vi "AutoBall.vi"(7 "Drive Params":T1, 8 "PID Params":T2, 10 "Command Array":dbl[](array[numeric])) -> (2 "isFinished":bool)   [LabVIEW 2013]
uses:
  AutoDriveParams.ctl
  Drivetrain/Drivetrain Control.ctl
  Drivetrain/DT Mode.ctl
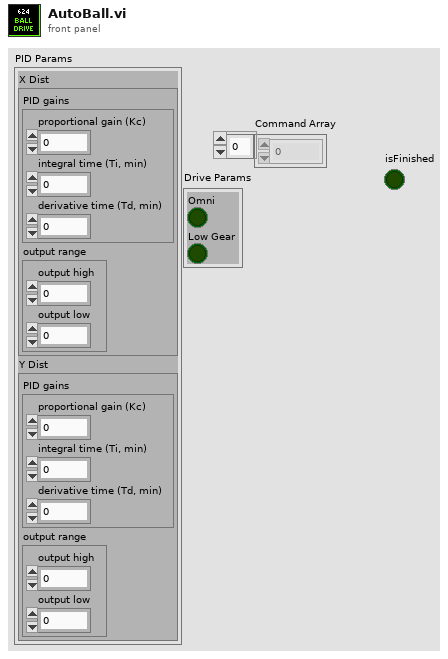
[diagram p1: front panel]
types:
  T1 = typedef "AutoDriveParams.ctl" = cluster{"Omni":bool, "Low Gear":bool}
  T2 = cluster{"X Dist":cluster{"PID gains":cluster{"proportional gain (Kc)":dbl, "integral time (Ti, min)":dbl, "derivative time (Td, min)":dbl}, "output range":cluster{"output high":dbl, "output low":dbl}}, "Y Dist":cluster{"PID gains":cluster{"proportional gain (Kc)":dbl, "integral time (Ti, min)":dbl, "derivative time (Td, min)":dbl}, "output range":cluster{"output high":dbl, "output low":dbl}}}
  T3 = typedef "DT Mode.ctl" = enum16{"Manual", "Gyro Steer", "Distance Drive", "Fieldcentric", "Roll Maneuver", "Alt Roll Maneuver"}
  T4 = typedef "Drivetrain Control.ctl" = cluster{"axis 1 (x)":dbl, "axis 2 (y)":dbl, "Mode":T3, "heading target":dbl, "steer axis":dbl, "omni?":bool, "Low Gear?":bool, "distance target":cluster{"x":dbl, "y":dbl}, "PID Params":cluster{"X Dist":cluster{"PID gains":cluster{"proportional gain (Kc)":dbl, "integral time (Ti, min)":dbl, "derivative time (Td, min)":dbl}, "output range":cluster{"output high":dbl, "output low":dbl}}, "Y Dist":cluster{"PID gains":cluster{"proportional gain (Kc)":dbl, "integral time (Ti, min)":dbl, "derivative time (Td, min)":dbl}, "output range":cluster{"output high":dbl, "output low":dbl}}}, "Coast":bool}
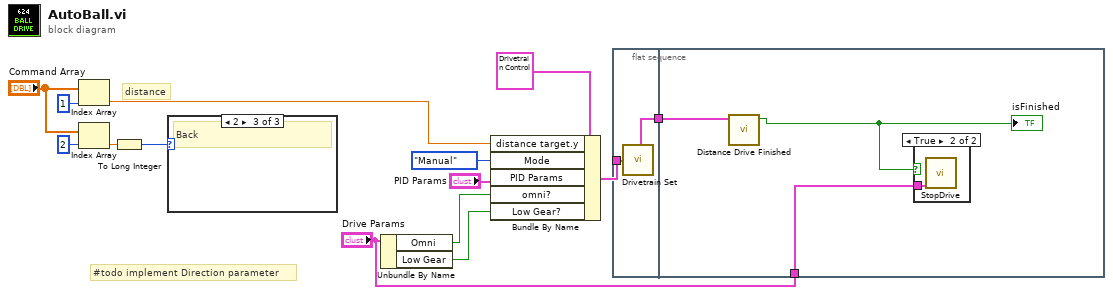
[diagram p0: block diagram]
diagram:
  # "#todo implement Direction parameter"
  # "distance"
  n1 = Index Array(array="Command Array", index=1) -> (element=w10:dbl)
  n2 = Index Array(array="Command Array", index=2) -> (element=w6:dbl)
  n3 = To Long Integer(number=w6) -> (32bit integer=w5:i32)
  n4 = case shown="2" w5 {
    frame 0, Default {
      # "Both"
    }
    frame 1 {
      # "Front"
    }
    frame 2 {
      # "Back"
    }
  }
  n5 = Unbundle By Name("Drive Params") -> ("Omni"=w4:bool, "Low Gear"=w3:bool)
  n6 = Bundle By Name(cluster=T4 {"axis 1 (x)"=0.0, "axis 2 (y)"=0.0, "Mode"=enum."Manual", "heading target"=0.0, "steer axis"=0.0, "omni?"=FALSE, "Low Gear?"=FALSE, "distance target"={"x"=0.0, "y"=0.0}, "PID Params"={"X Dist"={"PID gains"={"proportional gain (Kc)"=1.0, "integral time (Ti, min)"=0.0, "derivative time (Td, min)"=0.0}, "output range"={"output high"=1.0, "output low"=-1.0}}, "Y Dist"={"PID gains"={"proportional gain (Kc)"=1.0, "integral time (Ti, min)"=0.0, "derivative time (Td, min)"=0.0}, "output range"={"output high"=1.0, "output low"=-1.0}}}, "Coast"=FALSE} ("Drivetrain Control"), "distance target.y"=w10, "Mode"=DT_Mode."Manual", "PID Params"="PID Params", "omni?"=w4, "Low Gear?"=w3) -> (w7:T4)
  n7 = flat-sequence {
    tunnel: w7 -> [w15]
    tunnel: [w15] -> w1
    tunnel: "Drive Params" -> [w18]
    tunnel: w1 -> [w16]
    frame #0 {
      n8 = call "Drivetrain Set.vi"("Drivetrain Control"=w15) -> ()  [unwired: 1 in]
    }
    frame #1 {
      n9 = call "Distance Drive Finished.vi"("Drivetrain Control"=w16) -> ("Finished"=w17:bool)  [unwired: 10 in]
      "isFinished" <- w17
      n10 = case shown="True" w17 {
        tunnel: w18 -> [_ w19]
        frame False {
        }
        frame True {
          n11 = call "StopDrive.vi"("Drive Params"=w19) -> ()  [unwired: 11 in]
        }
      }
    }
  }
